vi "军蚁-模板匹配.vi"(0 "Image In":T9(plugin-control), 1 "Template File Path":path=path "C:/Users/hedongpo/Desktop/514-hdp/Alignment Assemble System/Source Code/Template Program/potteryTemplete/Temp3.png", 2 "Settings":T12={"Curve Parameters"={"Extraction Mode"=0, "Edge Threshold"=75, "Edge Filter Size"=1, "Min Length"=25, "Row Search Step Size"=15, "Col Search Step Size"=15, "Max Endpoint Gap"=10, "Closed"=FALSE, "Subpixel"=FALSE}, "Match Mode"={"Rotation"=TRUE, "Scale"=FALSE, "Occlusion"=TRUE, "Reserved"=FALSE, "Reserved"=FALSE, "Reserved"=FALSE}, "Range Settings"=[{"Match Constraints"=0, "Min"=0.0, "Max"=360.0}, {"Match Constraints"=2, "Min"=0.0, "Max"=25.0}], "Number of Matches"=1, "Minimum Match Score"=800.0, "SubPixel Accuracy"=FALSE, "Adv. Geometric Match Options 2"=[{"Setup Data Item"=21, "Item Value"=0.0}, {"Setup Data Item"=22, "Item Value"=1.0}]} {"Curve Parameters"."Extraction Mode" items=["Normal", "Uniform Regions"]; "Curve Parameters"."Edge Filter Size" items=["Fine", "Normal", "Contour Tracing"]; "Curve Parameters"."Max Endpoint Gap" min=0; "Curve Parameters"."Col Search Step Size" min=1 max=255 step=1; "Curve Parameters"."Row Search Step Size" min=1 max=255 step=1; "Curve Parameters"."Min Length" min=0; "Curve Parameters"."Edge Threshold" min=1 max=350 step=1; "Range Settings"."Max" format="%.2f"; "Range Settings"."Min" format="%.2f"; "Range Settings"."Match Constraints" items=["Rotation Angle (degrees)", "Scale Factor (%)", "Occlusion (%)"]; "Adv. Geometric Match Options 2"."Setup Data Item" items=["Curve Extraction Mode", "Curve Edge Threshold", "Curve Edge Filter Size", "Min Curve Length", "Curve Row Search Step Size", "Curve Col Search Step Size", "Curve Max Endpoint Gap", "Extract Closed Curves", "Enable Subpixel Curve Extraction", "Enable Correlation Score", "Enable Subpixel Accuracy", "Subpixel Iterations", "Subpixel Tolerance", "Initial Match List Length", "Enable Target Template Curve Score", "Min Match Separation Distance", "Min Match Separation Angle", "Min Match Separation Scale", "Max Match Overlap", "Enable Coarse Result", "Enable Calibration Support", "Enable Contrast Reversal", "Search Strategy", "Refinement Match Factor", "Subpixel Match Factor"]}, 3 "Rectangle":T2 {"Rotation" format="%.2f"; "Left" scale=0.0..1024.0; "Right" scale=0.0..1024.0}, 4 "抓边":T2 {"Rotation" format="%.2f"; "Left" scale=0.0..1024.0; "Right" scale=0.0..1024.0}, 5 "抓边Options":T8={"Search Direction"=3, "Edge Options"={"Edge Polarity"=0, "Kernel Size"=3, "Width"=3, "Minimum Edge Strength"=50.0, "Interpolation Type"=enum."Bilinear Fixed", "Data Processing Method"=enum."Average"}, "Show Search Area"=TRUE, "Show Search Lines"=TRUE, "Show Edges Found"=TRUE, "Show Result"=TRUE, "Search Area Color"=65280, "Search Lines Color"=255, "Edge Locations Color"=16776960, "Result Color"=16711680, "Overlay Group Name"=""} {"Search Direction" items=["Left to Right", "Right to Left", "Top to Bottom", "Bottom to Top"]; "Edge Options"."Edge Polarity" items=["All Edges", "Rising Edges", "Falling Edges"]; "Edge Options"."Minimum Edge Strength" format="%.2f"; "Edge Options"."Width" step=2; "Edge Options"."Kernel Size" step=2}, 6 "抓边Fit Options":T4={"Number of Lines"=1, "Type"=enum."First Edge Rake", "Min. Score"=10.0, "Max. Score"=1000.0, "Orientation"=0.0, "Angle Range"=45.0, "Angle Tolerance"=1.0, "Step Size"=64, "Min. SNR (db)"=0.0, "Min. Points (%)"=25.0, "Hough Iterations"=5} {"Min. Points (%)" min=0.0 max=100.0; "Min. SNR (db)" min=0.0; "Max. Score" min=0.0 max=1024.0; "Min. Score" min=0.0 max=1024.0 step=1.0}, 7 "error in":errorcluster) -> (20 "Image Out":T9(plugin-control), 22 "元素":T13 {"Correlation Score" format="%.2f"; "Target Template Curve Score" format="%.2f"; "Template Target Curve Score" format="%.2f"; "Bounding Box"."y" format="%.2f"; "Bounding Box"."x" format="%.2f"; "Position"."y" format="%.2f"; "Position"."x" format="%.2f"; "Score" format="%.2f"; "Scale" format="%.2f"; "Angle" format="%.2f"; "Occlusion %" format="%.2f"}, 27 "error out":errorcluster)   [LabVIEW 2017]
uses:
  <vilib>/vision/Pattern Matching.llb/IMAQ GM Match Report.ctl
  <vilib>/vision/Pattern Matching.llb/IMAQ Curve Parameters.ctl
  <vilib>/vision/Pattern Matching.llb/IMAQ Match Range Setting.ctl
  <vilib>/vision/Measure.llb/Edge Options.ctl
  <vilib>/vision/Measure.llb/Edge Polarity.ctl
  <vilib>/vision/Measure.llb/Straight Edge Options.ctl
  <vilib>/vision/Measure.llb/Straight Edge Process.ctl
  <vilib>/vision/NI_Vision_Development_Module.lvlib
  Global System.vi
panel:
  out "输出簇 2":T1
  out "输出簇":T1
  out "Angle (Pixel)":dbl
  out "Cluster":T3
  out "Bounding Box":cluster{"x":sgl, "y":sgl}[](array[cluster])
  out "Calibrated Matches":T13[](array[typedef]) {"Correlation Score" format="%.2f"; "Target Template Curve Score" format="%.2f"; "Template Target Curve Score" format="%.2f"; "Bounding Box"."y" format="%.2f"; "Bounding Box"."x" format="%.2f"; "Position"."y" format="%.2f"; "Position"."x" format="%.2f"; "Score" format="%.2f"; "Scale" format="%.2f"; "Angle" format="%.2f"; "Occlusion %" format="%.2f"}
  # "Range"
types:
  T1 = cluster{"Origin":cluster{"X":sgl, "Y":sgl}, "Angle (deg)":sgl, "Axis Reference":u32}
  T2 = typedef "IMAQ Rectangle" = cluster{"Left":i32, "Top":i32, "Right":i32, "Bottom":i32, "Rotation":dbl}
  T3 = cluster{"Point1 (Pixels)":cluster{"X":sgl, "Y":sgl}, "Point2 (Pixels)":cluster{"X":sgl, "Y":sgl}, "Point1 (Real-World)":cluster{"X":sgl, "Y":sgl}, "Point2 (Real-World)":cluster{"X":sgl, "Y":sgl}, "Angle (Pixel)":dbl, "Angle (Real-World)":dbl, "Score":dbl, "Straightness":dbl, "Average SNR (db)":dbl, "Calibration Valid":bool}
  T4 = typedef "Straight Edge Options.ctl" = cluster{"Number of Lines":i32, "Type":T5, "Min. Score":dbl, "Max. Score":dbl, "Orientation":dbl, "Angle Range":dbl, "Angle Tolerance":dbl, "Step Size":u32, "Min. SNR (db)":dbl, "Min. Points (%)":dbl, "Hough Iterations":i32}
  T5 = typedef "Straight Edge Process.ctl" = enum32{"First Edge Rake", "Best Edge Rake", "Hough Edge Rake", "First Edge Projection", "Best Edge Projection"}
  T6 = typedef "Edge Options.ctl" = cluster{"Edge Polarity":T7, "Kernel Size":u32, "Width":u32, "Minimum Edge Strength":sgl, "Interpolation Type":enum32{"Zero Order", "Bilinear", "Quadratic", "Cubic", "Bilinear Fixed"}, "Data Processing Method":enum32{"Average", "Median"}}
  T7 = typedef "Edge Polarity.ctl" = u32
  T8 = cluster{"Search Direction":u32, "Edge Options":T6, "Show Search Area":bool, "Show Search Lines":bool, "Show Edges Found":bool, "Show Result":bool, "Search Area Color":u32, "Search Lines Color":u32, "Edge Locations Color":u32, "Result Color":u32, "Overlay Group Name":string}
  T9 = typedef "IMAQ Image.ctl" = refnum<image>
  T10 = typedef "IMAQ Curve Parameters.ctl" = cluster{"Extraction Mode":u32, "Edge Threshold":i32, "Edge Filter Size":u32, "Min Length":i32, "Row Search Step Size":i32, "Col Search Step Size":i32, "Max Endpoint Gap":i32, "Closed":bool, "Subpixel":bool}
  T11 = typedef "IMAQ Match Range Setting.ctl" = cluster{"Match Constraints":u32, "Min":dbl, "Max":dbl}
  T12 = cluster{"Curve Parameters":T10, "Match Mode":cluster{"Rotation":bool, "Scale":bool, "Occlusion":bool, "Reserved":bool, "Reserved":bool, "Reserved":bool}, "Range Settings":T11[], "Number of Matches":i32, "Minimum Match Score":sgl, "SubPixel Accuracy":bool, "Adv. Geometric Match Options 2":cluster{"Setup Data Item":u16, "Item Value":dbl}[]}
  T13 = typedef "IMAQ GM Match Report.ctl" = cluster{"Position":cluster{"x":sgl, "y":sgl}, "Angle":sgl, "Scale":sgl, "Score":sgl, "Bounding Box":cluster{"x":sgl, "y":sgl}[], "Contrast Reversed":bool, "Occlusion %":sgl, "Template Target Curve Score":sgl, "Target Template Curve Score":sgl, "Correlation Score":sgl}
  T14 = enum16{"Reset", "Update Coordinate System", "Get Coordinate System"}
  T15 = enum16{"Horizontal Motion", "Vertical Motion", "Horizontal and Vertical Motion", "Horizontal, Vertical and Angular Motion"}
  T16 = cluster{"Desired Font (Application)":enum16{"User-specified Font", "Application Font", "System Font", "Dialog Font"}, "[User-specified Font]":cluster{"Font Name":string, "Size":i16, "Strikeout?":bool, "Italic?":bool, "Underline?":bool, "Outline?":bool, "Shadow?":bool, "Bold?":bool, "Rotation Angle":dbl}, "Horizontal Alignment":i16, "Vertical Alignment":i16}
  T17 = cluster{"Global Rectangle":i32[], "Contours":cluster{"ID":enum32{"External", "Internal"}, "Type":u32, "Coordinates":i32[]}[]}
  T18 = typedef "ROI Descriptor" = cluster{"Global Rectangle":i32[], "Contours":cluster{"ID":enum32{"External", "Internal"}, "Type":u32, "Coordinates":i32[]}[]}
  T19 = typedef "IMAQ Coordinate System" = cluster{"Reference System":cluster{"Origin":cluster{"X":sgl, "Y":sgl}, "Angle (deg)":sgl, "Axis Reference":u32}, "Measurement System":cluster{"Origin":cluster{"X":sgl, "Y":sgl}, "Angle (deg)":sgl, "Axis Reference":u32}}
  T20 = cluster{"Point1 (Pixels)":cluster{"X":sgl, "Y":sgl}, "Point2 (Pixels)":cluster{"X":sgl, "Y":sgl}, "Point1 (Real-World)":cluster{"X":sgl, "Y":sgl}, "Point2 (Real-World)":cluster{"X":sgl, "Y":sgl}, "Angle (Pixel)":dbl, "Angle (Real-World)":dbl, "Score":dbl, "Straightness":dbl, "Average SNR (db)":dbl, "Calibration Valid":bool}[]
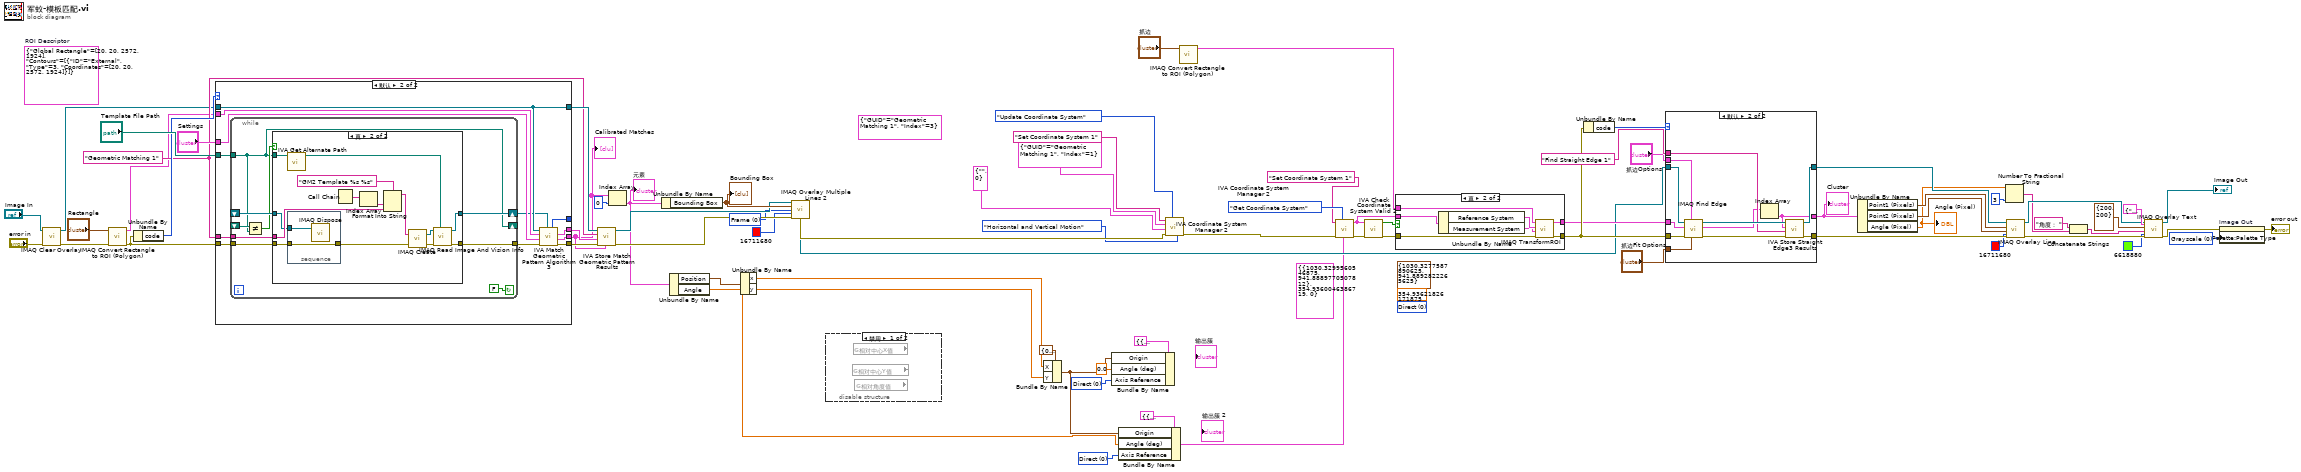
[diagram p0: block diagram]
diagram:
  w4 = u32 0 items=["Direct", "Indirect"] ("Axis Reference")
  (unwired) cluster{"GUID":string, "Index":i32} {"GUID"="Geometric Matching 1", "Index"=3} ("Angle ID")
  (unwired) T1 {"Origin"={"X"=1030.33, "Y"=941.889}, "Angle (deg)"=354.936, "Axis Reference"=0} ("Reference System")
  (unwired) cluster{"X":sgl, "Y":sgl} {"X"=1030.3278, "Y"=941.8893} ("Origin")
  (unwired) sgl 354.93622 ("Angle (deg)")
  (unwired) u32 0 items=["Direct", "Indirect"] ("Axis Reference")
  w40 = u32 0 items=["Direct", "Indirect"] ("Axis Reference")
  w62 = u32 0 items=["Frame", "Fill"] ("Drawing Mode (Frame)")
  w68 = u32 0 items=["Grayscale", "Binary", "Gradient", "Rainbow", "Temperature", "User Defined", "Binary 16 Bit", "Gradient 16 Bit", "Rainbow 16 Bit", "Temperature 16 Bit", "User Defined 16 Bit"] ("Palette Type")
  w70 = "Geometric Matching 1" ("Step Name")
  (unwired) T17 {"Global Rectangle"=[20, 20, 2572, 1924], "Contours"=[{"ID"=enum."External", "Type"=3, "Coordinates"=[20, 20, 2572, 1924]}]}  # ROI Descriptor
  n1 = call "IMAQ Clear Overlay"("error in (no error)"="error in", "Image"="Image In") -> ("error out"=w56:errorcluster, "Image Out"=w54:T9)  [unwired: 8 in]
  n2 = call "IMAQ Convert Rectangle to ROI (Polygon)"("error in (no error)"=w56, "Rectangle"="Rectangle") -> ("error out"=w59:errorcluster, "ROI Descriptor"=w58:T18)  [unwired: 6 in, 1 out]
  n3 = Unbundle By Name(w59) -> ("code"=w73:i32)
  n4 = case "条件结构" shown="默认" w73 {
    tunnel: "Template File Path" -> [_ w79]
    tunnel: w59 -> [_ w80]
    tunnel: "Settings" -> [_ w89]
    tunnel: w58 -> [_ w88]
    tunnel: w54 -> [w77 w83]
    tunnel: [_ w87] -> w75
    tunnel: [_ w86] -> w74
    tunnel: [_ w85] -> w67
    tunnel: [_ w84] -> _
    tunnel: [w77 w83] -> w72
    tunnel: w70 -> [_ w78]
    frame -1074396199, -1074396198 {
      # "Discard Coordinate System Error"
    }
    frame Default {
      n5 = while {
        shift-right: [w98] -> w81
        shift-left: _ -> [w97]
        tunnel: [w95] -> w82
        tunnel: w80 -> [w94]
        tunnel: w79 -> [w90]
        tunnel: w78 -> [w93]
        shift-right: [w90] -> _
        shift-left: _ -> [w92]
        stop <- FALSE continue-if-true
        n6 = Not Equal?(x=w92, y=w90) -> (x != y?=w91:bool)
        n7 = case "条件结构" shown="真" w91 {
          tunnel: [w100 w112] -> w98
          tunnel: w97 -> [w100 w104]
          tunnel: [w99 w109] -> w95
          tunnel: w94 -> [w99 w105]
          tunnel: w93 -> [_ w106]
          tunnel: w90 -> [_ w102]
          frame False {
          }
          frame True {
            n8 = call <vilib>:"IVA Get Alternate Path.vi"("Path In"=w102) -> ("Path Out"=w101:path)  [unwired: 10 out]
            n9 = stacked-sequence "层叠式顺序结构" {
              tunnel: w105 -> [w116]
              tunnel: w104 -> [w115]
              tunnel: [w116] -> w103
              frame #0 {
                n10 = call "IMAQ Dispose"("Image"=w115) -> ()  [unwired: 2 in, 4 out]
              }
            }
            n11 = Call Chain() -> (call chain=w108:string[])
            n12 = Index Array(array=w108) -> (element=w107:string)  [unwired: 1 in]
            n13 = Format Into String(format string="GM2 Template %s %s" ("Image Name"), w107, w106) -> (resulting string=w114:string)  [unwired: 2 in, 1 out]
            n14 = call "IMAQ Create"("Image Name"=w114, "error in (no error)"=w103) -> ("New Image"=w111:T9, "error out"=w110:errorcluster)  [unwired: 2 in, 1 out]
            n15 = call "IMAQ Read Image And Vision Info"("File Path"=w101, "error in (no error)"=w110, "Image"=w111) -> ("error out"=w109:errorcluster, "Image Out"=w112:T9)  [unwired: 1 in, 6 out]
          }
        }
      }
      n16 = call <vilib>:"IVA Match Geometric Pattern Algorithm 3.vi"("Template"=w81, "error in (no error)"=w82, "Settings"=w89, "ROI Descriptor"=w88, "Image"=w83) -> ("error out"=w87:errorcluster, "Calibrated Matches"=w85:T13[], "Matches"=w86:T13[], "Number of Matches"=w84:i32)  [unwired: 3 out]
    }
  }
  "Calibrated Matches" <- w67
  n17 = call <vilib>:"IVA Store Match Geometric Pattern Results.vi"("Calibrated Matches"=w67, "error in (no error)"=w75, "Matches"=w74, "Step Name"=w70, "Image in"=w72) -> ("error out"=w63:errorcluster, "Image dup"=w64:T9)  [unwired: 5 out]
  n18 = Index Array(array=w67, index=0 ("索引")) -> (element=w10:T13)
  "元素" <- w10
  n19 = Unbundle By Name(w10) -> ("Bounding Box"=w65:cluster{"x":sgl, "y":sgl}[])
  "Bounding Box" <- w65
  n20 = Unbundle By Name(w10) -> ("Position"=w9:cluster{"x":sgl, "y":sgl}, "Angle"=w2:sgl)
  n21 = Unbundle By Name(w9) -> ("x"=w8:sgl, "y"=w7:sgl)
  n22 = call "IMAQ Overlay Multiple Lines 2"("Image"=w64, "Line End Points"=w65, "Drawing Mode (Frame)"=w62, "Color"=u32 16711680, "error in (no error)"=w63) -> ("Image Out"=w17:T9, "error out"=w22:errorcluster)  [unwired: 9 in]
  n23 = disable-structure shown="禁用" {
    frame Disabled {
      n24 = global read "Global System.vi" "相对中心Y值"() -> ()  [unwired: 1 out]
      n25 = global read "Global System.vi" "相对中心X值"() -> ()  [unwired: 1 out]
      n26 = global read "Global System.vi" "相对角度值"() -> ()  [unwired: 1 out]
    }
    frame Enabled {
    }
  }
  n27 = Bundle By Name(cluster=cluster{"X":sgl, "Y":sgl} {"X"=0.0, "Y"=0.0} ("Origin"), "X"=w8, "Y"=w7) -> (w3:cluster{"X":sgl, "Y":sgl})
  n28 = Bundle By Name(cluster=T1 {"Origin"={"X"=0.0, "Y"=0.0}, "Angle (deg)"=0.0, "Axis Reference"=0} ("Reference System"), "Origin"=w3, "Angle (deg)"=sgl 0.0, "Axis Reference"=w40) -> ()  [unwired: 1 out]
  n29 = Bundle By Name(cluster=T1 {"Origin"={"X"=0.0, "Y"=0.0}, "Angle (deg)"=0.0, "Axis Reference"=0} ("Reference System"), "Origin"=w3, "Angle (deg)"=w2, "Axis Reference"=w4) -> (w1:T1)
  n30 = call <vilib>:"IVA Coordinate System Manager 2.vi"("Mode"=T15."Horizontal and Vertical Motion", "Function"=T14."Update Coordinate System", "error in (no error)"=w22, "Angle ID"=cluster{"GUID":string, "Index":i32} {"GUID"="", "Index"=0}, "Origin ID"=cluster{"GUID":string, "Index":i32} {"GUID"="Geometric Matching 1", "Index"=1}, "Coordinate System Name"="Set Coordinate System 1") -> ("error out"=w16:errorcluster)  [unwired: 1 in, 4 out]
  n31 = call "IMAQ Convert Rectangle to ROI (Polygon)"("Rectangle"="抓边") -> ("ROI Descriptor"=w18:T18)  [unwired: 7 in, 2 out]
  n32 = call <vilib>:"IVA Coordinate System Manager 2.vi"("Reference System"=w1, "Function"=T14."Get Coordinate System", "error in (no error)"=w16, "Coordinate System Name"="Set Coordinate System 1") -> ("error out"=w51:errorcluster, "Coordinate System Out"=w49:T19)  [unwired: 3 in, 3 out]
  n33 = call <vilib>:"IVA Check Coordinate System Valid 2.vi"("error in (no error)"=w51, "Coordinate System"=w49) -> ("error out"=w47:errorcluster, "Valid?"=w48:bool)  [unwired: 8 out]
  n34 = case "条件结构" shown="真" w48 {
    tunnel: w18 -> [w118 w125]
    tunnel: [w118 w122] -> w46
    tunnel: [w117 w121] -> w50
    tunnel: w49 -> [_ w120]
    tunnel: w47 -> [w117 w119]
    frame False {
    }
    frame True {
      n35 = Unbundle By Name(w120) -> ("Reference System"=w124:T1, "Measurement System"=w123:T1)
      n36 = call "IMAQ TransformROI"("error in (no error)"=w119, "New Reference"=w123, "Base Reference"=w124, "ROI Descriptor"=w125) -> ("error out"=w121:errorcluster, "ROI Descriptor out"=w122:T18)  [unwired: 6 out]
    }
  }
  n37 = Unbundle By Name(w50) -> ("code"=w44:i32)
  n38 = case "条件结构" shown="默认" w44 {
    tunnel: w17 -> [w126 w138]
    tunnel: w50 -> [_ w137]
    tunnel: w46 -> [_ w131]
    tunnel: [w126 w135] -> w37
    tunnel: [_ w133] -> w36
    tunnel: "Find Straight Edge 1" ("Step Name") -> [_ w132]
    tunnel: "抓边Fit Options" -> [_ w130]
    tunnel: "抓边Options" -> [_ w129]
    tunnel: [_ w127] -> w38
    frame -1074396199, -1074396198 {
      # "Discard Coordinate System Error"
    }
    frame Default {
      n39 = call "IMAQ Find Edge"("Line Fit Options"=w130, "Options"=w129, "error in (no error)"=w137, "ROI Descriptor"=w131, "Image"=w138) -> ("error out"=w134:errorcluster, "Straight Edges"=w128:T20, "Image Out"=w136:T9)  [unwired: 1 in, 3 out]
      n40 = Index Array(array=w128) -> (element=w127:T3)  [unwired: 1 in]
      n41 = call <vilib>:"IVA Store Straight Edge3 Results.vi"("error in (no error)"=w134, "Step Name"=w132, "Straight Edge"=w127, "Image in"=w136) -> ("error out"=w133:errorcluster, "Image dup"=w135:T9)  [unwired: 1 in, 5 out]
    }
  }
  "Cluster" <- w38
  n42 = Unbundle By Name(w38) -> ("Point1 (Pixels)"=w35:cluster{"X":sgl, "Y":sgl}, "Point2 (Pixels)"=w34:cluster{"X":sgl, "Y":sgl}, "Angle (Pixel)"=w28:dbl)
  "Angle (Pixel)" <- w28
  n43 = Number To Fractional String(number=w28, precision (6)=i16 3 ("精度(6)")) -> (F-format string=w25:string)  [unwired: 2 in]
  n44 = call "IMAQ Overlay Line"("Color"=u32 16711680, "error in (no error)"=w36, "End Point"=w34, "Start Point"=w35, "Image"=w37) -> ("error out"=w29:errorcluster, "Image Out"=w30:T9)  [unwired: 5 in]
  n45 = Concatenate Strings("角度： " ("字符串"), w25) -> (w24:string)
  n46 = call "IMAQ Overlay Text"("Text Color (black)"=u32 6618880, "Font, Size & Style"=T16 {"Desired Font (Application)"=enum."User-specified Font", "[User-specified Font]"={"Font Name"="", "Size"=100, "Strikeout?"=FALSE, "Italic?"=FALSE, "Underline?"=FALSE, "Outline?"=FALSE, "Shadow?"=FALSE, "Bold?"=TRUE, "Rotation Angle"=0.0}, "Horizontal Alignment"=0, "Vertical Alignment"=0}, "error in (no error)"=w29, "String"=w24, "Origin"=cluster{"X":i32, "Y":i32} {"X"=200, "Y"=200}, "Image"=w30) -> ("error out"=w20:errorcluster, "Image Out"=→"Image Out":T9)  [unwired: 4 in]
  n47 = property on="Image Out" class="ImageControl"(error in=w20, "Palette:Palette Type"=w68) -> (error out=→"error out":errorcluster)  [unwired: 1 in, 1 out]
